vi "getOffsetToUTC.vi"(11 "Epoch (UNIX)":refnum<class "Epoch.UNIX.lvclass">) -> (2 "Offset to UTC":i64)   [LabVIEW 2021, in "Epoch.UNIX.lvclass"]
uses:
  Epoch.UNIX.lvclass
  Epoch.UNIX.lvclass/Epoch.UNIX.ctl
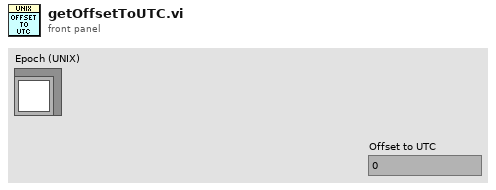
[diagram p1: front panel]
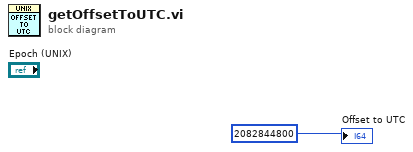
[diagram p0: block diagram]
diagram:
  "Offset to UTC" <- i64 2082844800 ("Timestamp Offset")
